vi "ReadSize.vi"(8 "error in (no error)":errorcluster, 11 "reference in":refnum<class "Pgui_Obj.lvclass">) -> (0 "error out":errorcluster, 2 "Size":cluster{"Width":i16, "Height":i16}, 3 "reference out":refnum<class "Pgui_Obj.lvclass">)   [LabVIEW 2019, in "Pgui_Obj.lvclass"]
doc: "Sets Width And height of object"
uses:
  Pgui_Obj.lvclass
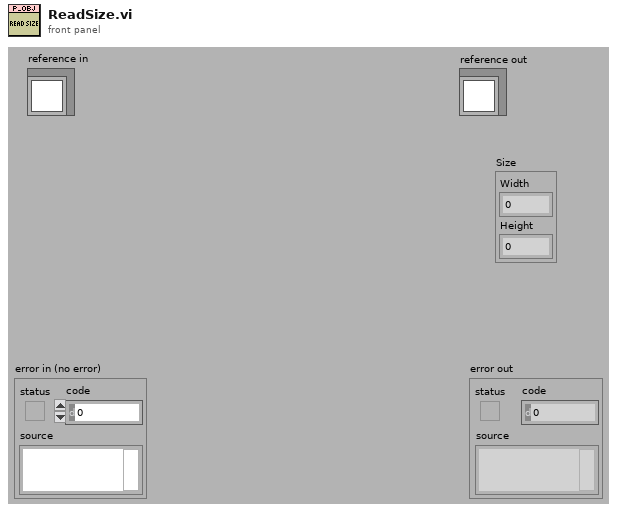
[diagram p1: front panel]
types:
  T1 = typedef "Pgui_Obj.lvclass/ObjectAttributes.ctl" = cluster{"Children":refnum<class "Pgui_Obj.lvclass">[], "Draw Instr":picture, "Params":cluster{"left":i16, "top":i16, "right":i16, "bottom":i16}, "Parent_Pgui_Obj":refnum<class "Pgui_Obj.lvclass">, "MouseOver":bool}
  T2 = cluster{"left":i16, "top":i16, "right":i16, "bottom":i16}
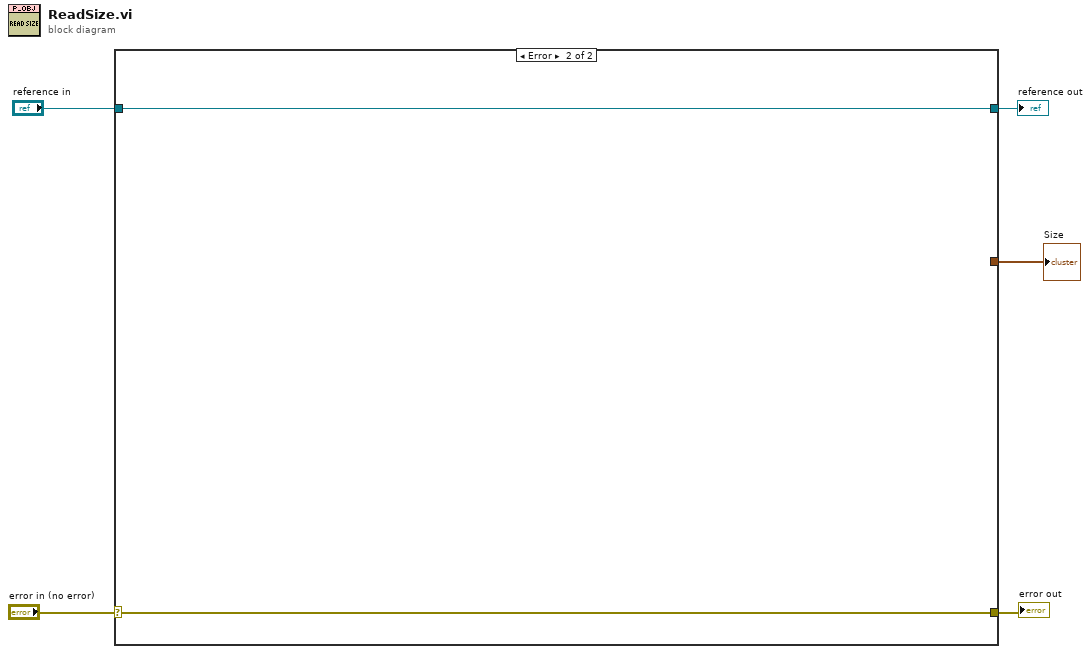
[diagram p0: block diagram]
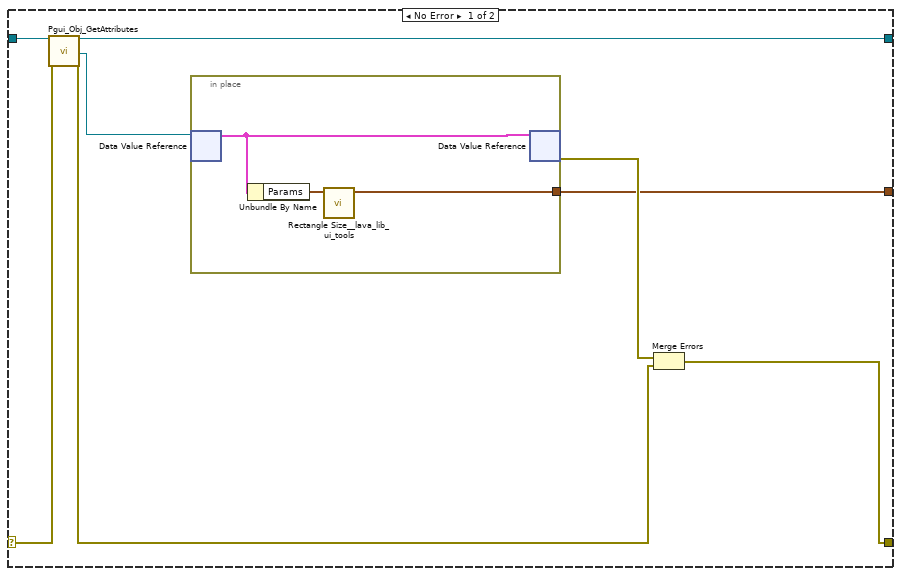
[diagram p2: hidden frame]
diagram:
  n1 = case shown="Error" "error in (no error)" {
    selector: "error in (no error)" -> [w13 w18]
    tunnel: [w8 w18] -> w4
    tunnel: [w11 w17] -> w2
    tunnel: "reference in" -> [w12 w17]
    tunnel: [w6 _] -> w1
    frame No Error {
      n2 = call "Pgui_Obj_GetAttributes.vi"("reference in"=w12, "error in (no error)"=w13) -> ("reference out"=w11:refnum<class "Pgui_Obj.lvclass">, "DataRef"=w7:refnum<data-value>, "error out"=w9:errorcluster)  [unwired: 14 in, 1 out]
      n3 = in-place {
        in-place-border: [w14] -> w6
        n4 = in-place-dvr #1(w7) -> (w16:T1)  [unwired: 1 out]
        n5 = Unbundle By Name(w16) -> ("Params"=w15:T2)
        n6 = call <vilib>:"Rectangle Size__lava_lib_ui_tools.vi"("Rectangle"=w15) -> ("Rect Size"=w14:cluster{"width":i32, "height":i32})  [unwired: 8 in, 2 out]
        n7 = in-place-dvr #1(w16) -> (w10:errorcluster)  [unwired: 1 out]
      }
      n8 = Merge Errors(w10, w9) -> (w8:errorcluster)
    }
    frame Error {
    }
  }
  "error out" <- w4
  "reference out" <- w2
  "Size" <- w1
